vi "Cargo Arm Encoder Input.vi"() -> (0 "Cargo Arm Distance (cm)":dbl)   [LabVIEW 2018]
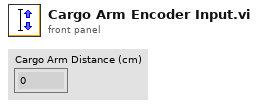
[diagram p1: front panel]
types:
  T1 = typedef "WPI_PotentiometerDevRef.ctl" = cluster{"DevStatus":errorcluster, "Analog Channel":T2, "Invert Output":bool}
  T2 = typedef "FPGA_AIChannel.ctl" = enum8{"AI 0", "AI 1", "AI 2", "AI 3", "AI MXP 0", "AI MXP 1", "AI MXP 2", "AI MXP 3", "Invalid"}
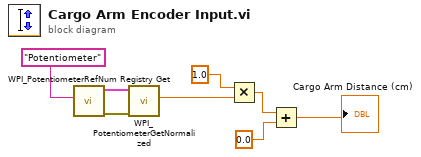
[diagram p0: block diagram]
diagram:
  n1 = call <vilib>:"WPI_PotentiometerRefNum Registry Get.vi"("refnum name"="Potentiometer") -> ("error out"=w8:errorcluster, "PotDevRef"=w7:T1)  [unwired: 9 in]
  n2 = call <vilib>:"WPI_PotentiometerGetNormalized.vi"("error in"=w8, "PotDevRef"=w7) -> ("Normalized Value"=w5:dbl)  [unwired: 7 in, 2 out]
  n3 = Multiply(x=1.0, y=w5) -> (x*y=w3:dbl)
  n4 = Add(x=w3, y=0.0) -> (x+y=→"Cargo Arm Distance (cm)":dbl)
